vi "class variable.vi"() -> ()   [LabVIEW 2012, in "DAQOrcaFlash.lvclass"]
uses:
  DAQOrcaFlash.lvclass
panel:
  in  "terminate?":bool
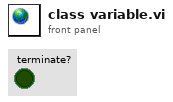
[diagram p1: front panel]
diagram:
